vi "UART Read.vi"(5 "error in (no error)":errorcluster, 6 "TimeOut(s)":dbl=3.0, 7 "ExpectStr":string="OK", 8 "VISA Resource In":refnum<visa-resource-name>="COM1") -> (0 "error out":errorcluster, 1 "OK?":bool, 2 "StrOut":string, 3 "VISA Resource Out":refnum<visa-resource-name>)   [LabVIEW 2015]
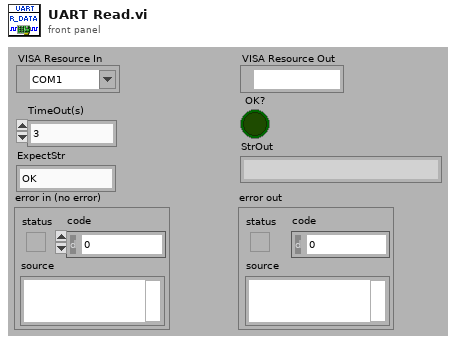
[diagram p1: front panel]
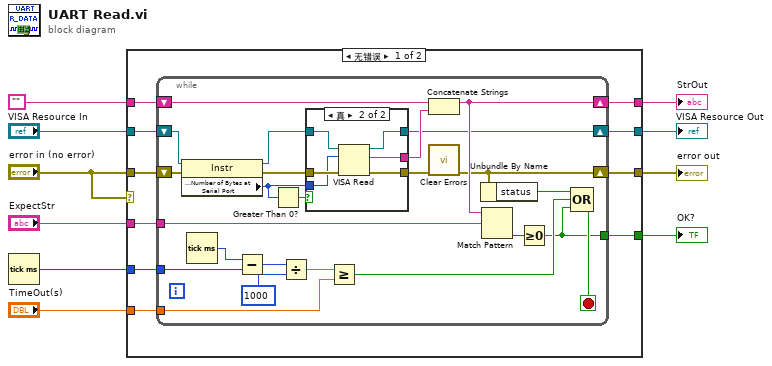
[diagram p0: block diagram]
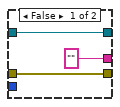
[diagram p2: hidden frame]
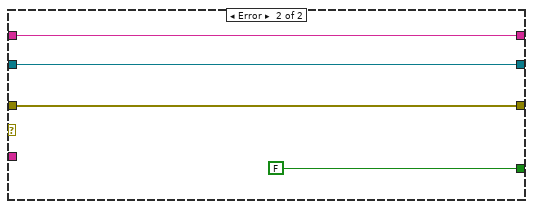
[diagram p3: hidden frame]
diagram:
  n1 = Tick Count (ms)() -> (millisecond timer value=w9:u32)
  n2 = case shown="无错误" "error in (no error)" {
    tunnel: "" -> [w20 w54]
    tunnel: w9 -> [w19 _]
    tunnel: "VISA Resource In" -> [w18 w57]
    tunnel: "error in (no error)" -> [w17 w56]
    tunnel: "ExpectStr" -> [w16 _]
    tunnel: [w15 w54] -> w6
    tunnel: [w14 w56] -> w5
    tunnel: [w13 w57] -> w4
    tunnel: "TimeOut(s)" -> [w12 _]
    tunnel: [w11 FALSE] -> w2
    frame No Error {
      n3 = while {
        shift-right: [w21] -> w14
        shift-left: w17 -> [w42]
        shift-right: [w37] -> w15
        shift-left: w20 -> [w39]
        tunnel: w19 -> [w35]
        tunnel: w12 -> [w24]
        tunnel: w16 -> [w26]
        shift-right: [w25] -> w13
        shift-left: w18 -> [w29]
        tunnel: [w22] -> w11
        stop <- w30 stop-if-true
        n4 = property class="Instr"(reference=w29, error in=w42) -> (reference out=w43:refnum<visa-resource-name>, error out=w41:errorcluster, "Serial Settings:Number of Bytes at Serial Port"=w40:u32)
        n5 = Tick Count (ms)() -> (millisecond timer value=w36:u32)
        n6 = Subtract(x=w36, y=w35) -> (x-y=w27:u32)
        n7 = Greater Than 0?(x=w40) -> (x > 0?=w44:bool)
        n8 = Divide(x=w27, y=u32 1000) -> (x/y=w34:dbl)
        n9 = case shown="真" w44 {
          tunnel: w43 -> [w45 w53]
          tunnel: w41 -> [w47 w52]
          tunnel: w40 -> [_ w51]
          tunnel: [w47 w50] -> w33
          tunnel: [w45 w49] -> w25
          tunnel: ["" ("read buffer") w48] -> w38
          frame False {
          }
          frame True {
            n10 = VISA Read(VISA resource name=w53, byte count=w51, error in (no error)=w52) -> (VISA resource name out=w49:refnum<visa-resource-name>, read buffer=w48:string, error out=w50:errorcluster)  [unwired: 1 out]
          }
        }
        n11 = Greater Or Equal?(x=w34, y=w24) -> (x >= y?=w23:bool)
        n12 = Concatenate Strings(w39, w38) -> (w37:string)
        n13 = call <vilib>:"Clear Errors.vi"("error in (no error)"=w33) -> ("error out"=w21:errorcluster)  [unwired: 5 in, 1 out]
        n14 = Unbundle By Name(w21) -> ("status"=w31:bool)
        n15 = Match Pattern(string=w37, regular expression=w26) -> (offset past match=w32:i32)  [unwired: 1 in, 3 out]
        n16 = Greater Or Equal To 0?(x=w32) -> (x >= 0?=w22:bool)
        n17 = Compound Arithmetic op=OR(w31, w23, w22) -> (w30:bool)
      }
    }
    frame Error {
    }
  }
  "StrOut" <- w6
  "VISA Resource Out" <- w4
  "error out" <- w5
  "OK?" <- w2
